vi "Autonomous Independent.vi"   [LabVIEW 2014]
doc: "This VI is called when autonomous begins, and will automatically be terminated when autonomous ends. You can carry out timed or sensor driven robot movement independently without needing to return to the caller."
uses:
  <vilib>/Rock Robotics/WPI/Joystick/WPI_JoystickGetSetRefNum.vi
  <vilib>/Rock Robotics/Network Tables/SD Write Numeric Array.vi
  Robot Global Data.vi
  <vilib>/addons/control/pid/pid.llb/PID (DBL).vi
  navX-MXP Library/navX-MXP IMU.lvlib
  <vilib>/addons/control/pid/NI_PID_pid.lvlib
panel:
  # "Be sure to right-click and choose Data Operations>>Make Current Value default if you want to save the array values with the VI"
types:
  T1 = cluster{"proportional gain (Kc)":dbl, "integral time (Ti, min)":dbl, "derivative time (Td, min)":dbl}
  T2 = typedef "WPI_JoystickDevRef.ctl" = cluster{"Device":T3}
  T3 = typedef "WPI_JoystickDeviceEnum.ctl" = enum16{"USB 0", "USB 1", "USB 2", "USB 3", "USB 4", "USB 5"}
  T4 = enum16{"centered", "deg0", "deg45", "deg90", "deg135", "deg180", "deg225", "deg270", "deg315"}
  T5 = typedef "WPI_MotorControlDeviceRef.ctl" = cluster{"DeviceStatus":errorcluster, "Type":T6, "PWM":cluster{"Controller":T7, "PWM Channel":T8, "DeadBand":T9}, "CAN":cluster{"Device Number":u8, "Control Mode":T10, "Semaphore":T11, "Max Vout":dbl, "TalonSRX Control Mode":T12}, "Invert":bool, "TransformRef":T13, "InvTransformRef":T13}
  T6 = typedef "WPI_MotorControlType.ctl" = enum16{"PWM", "CAN", "CANTalonSRX"}
  T7 = typedef "FPGA_TypedefDigitalModule.ctl" = enum16{"Controller 1"}
  T8 = typedef "FPGA_DIOPWMChannel.ctl" = enum8{"PWM 0", "PWM 1", "PWM 2", "PWM 3", "PWM 4", "PWM 5", "PWM 6", "PWM 7", "PWM 8", "PWM 9", "PWM MXP 0", "PWM MXP 1", "PWM MXP 2", "PWM MXP 3", "PWM MXP 4", "PWM MXP 5", "PWM MXP 6", "PWM MXP 7", "PWM MXP 8", "PWM MXP 9", "Invalid"}
  T9 = typedef "WPI_PWMDeadband.ctl" = cluster{"Name":string, "maxPositivePwm":i32, "minPositivePwm":i32, "centerPwm":i32, "maxNegativePwm":i32, "minNegativePwm":i32, "angularRange":u16}
  T10 = typedef "WPI_CANJaguar_ControlMode.ctl" = enum8{"Percent VBus", "Current", "Speed", "Position", "Voltage"}
  T11 = typedef "Semaphore RefNum" = refnum<k1>
  T12 = typedef "WPI_CANTalonSRX_APIControlMode.ctl" = enum8{"Percent VBus", "Speed", "Position", "Slave", "Unchanged / Invalid"}
  T13 = typedef "WPI_PWMTransform_ConPane.ctl" = refnum<vi>
  T14 = typedef "navX-MXP IMU.lvlib/navX Device TypeDef.ctl" = cluster{"navX Interface Protocol":T15, "navX Interface Protocol TypeDefs":cluster{"SPIDevRef":T16, "I2CDevRef":T18}, "navX System Information":cluster{"Board Information":T20, "Status":T21, "Offsets":T25}, "navX Common Information":cluster{"Update Rate (4Hz-60Hz)":T26, "refnum name":string, "error":errorcluster}}
  T15 = typedef "navX-MXP IMU.lvlib/navX Interface Protocol.ctl" = enum16{"SPI", "I2C"}
  T16 = typedef "WPI_SPIDevRef.ctl" = cluster{"DevStatus":errorcluster, "Handle":i32, "Controller":T7, "SPI Bus":T17}
  T17 = typedef "spi_bus.ctl" = enum16{"SPI On-Board, CS0", "SPI On-Board, CS1", "SPI On-Board, CS2", "SPI On-Board, CS3", "SPI MXP", "Invalid"}
  T18 = typedef "WPI_I2CDevRef.ctl" = cluster{"DevStatus":errorcluster, "Controller":T7, "Device Address":u8, "Handle":i32, "I2C Bus":T19}
  T19 = typedef "i2c_bus.ctl" = enum16{"I2C On-Board", "I2C MXP", "Invalid"}
  T20 = typedef "navX-MXP IMU.lvlib/navX Board Information.ctl" = cluster{"WhoAmI (50 | 0x32)":u8, "Board Revision":u8, "Firmware Major Version":u8, "Firmware Minor Version":u8}
  T21 = typedef "navX-MXP IMU.lvlib/navX Status Data.ctl" = cluster{"Update Rate Hz":u8, "Accelerometer Full-Scale Range":u8, "Gyro Full-Scale Range":u16, "NAVX_OP_STATUS":T22, "NAVX_CAL_STATUS":T23, "NAVX_SELFTEST_STATUS":u8, "NAVX_SENSOR_STATUS":T24}
  T22 = typedef "navX-MXP IMU.lvlib/navX NAVX_OP_STATUS.ctl" = u8
  T23 = typedef "navX-MXP IMU.lvlib/navX NAVX_CAL_STATUS.ctl" = u8
  T24 = typedef "navX-MXP IMU.lvlib/navX NAVX_SENSOR_STATUS.ctl" = cluster{"MOVING":bool, "YAW_STABLE":bool, "MAG_DISTURBANCE":bool, "ALTITUDE_VALID":bool, "SEALEVEL_PRESS_SET":bool, "FUSED_HEADING_VALID":bool}
  T25 = typedef "navX-MXP IMU.lvlib/navX Offsets Data.ctl" = cluster{"Yaw":dbl, "Quat W":dbl, "Quat X":dbl, "Quat Y":dbl, "Quat Z":dbl}
  T26 = typedef "navX-MXP IMU.lvlib/navX Update Rate.ctl" = u8
  T27 = typedef "navX-MXP IMU.lvlib/navX YPRH Data.ctl" = cluster{"Yaw":dbl, "Pitch":dbl, "Roll":dbl, "Heading":dbl}
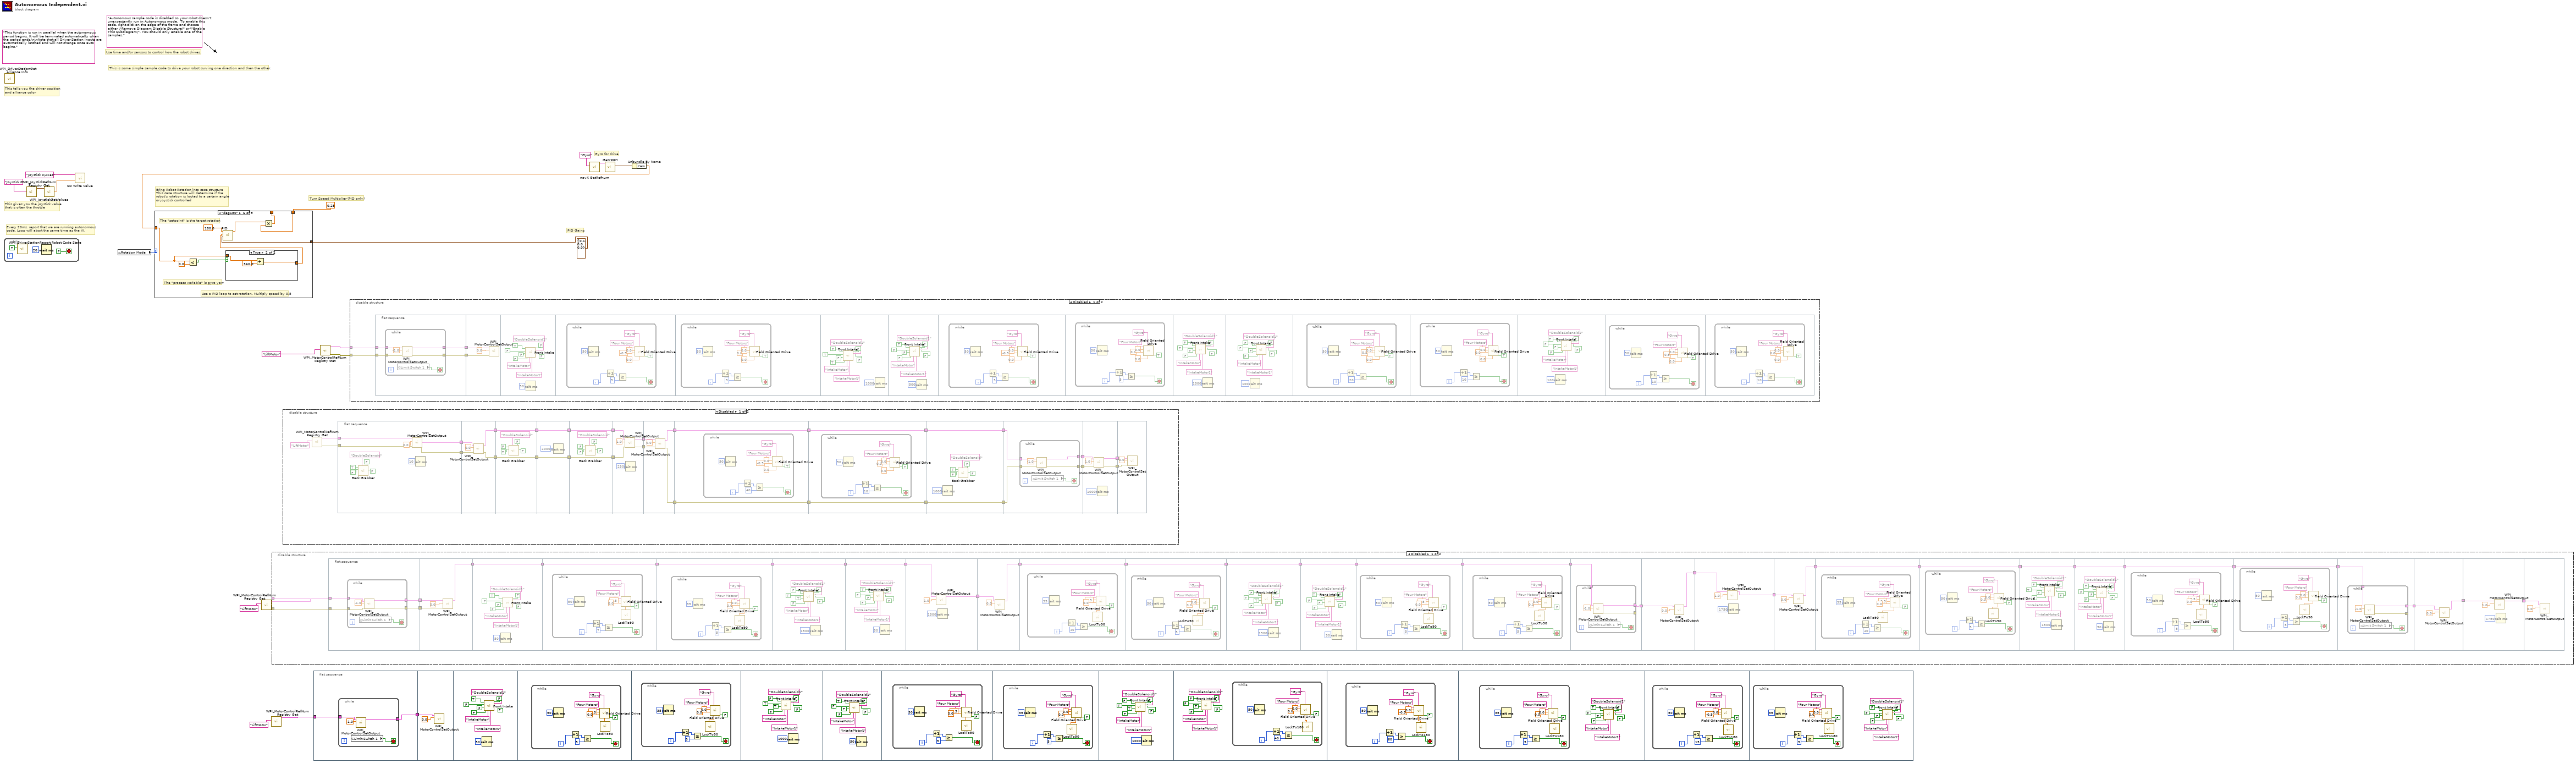
[diagram p0: block diagram]
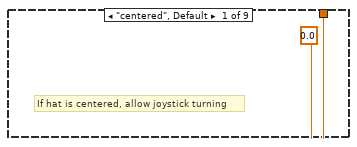
[diagram p5: hidden frame]
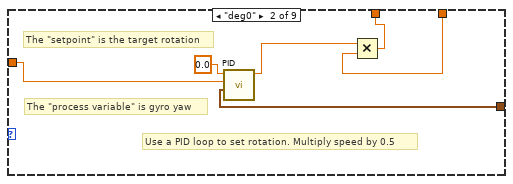
[diagram p6: hidden frame]
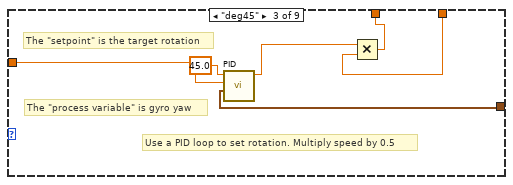
[diagram p7: hidden frame]
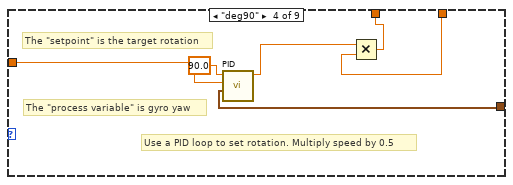
[diagram p8: hidden frame]
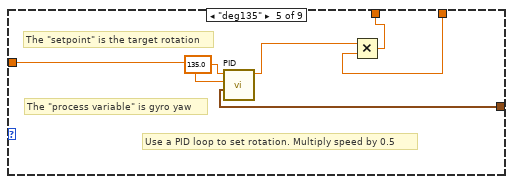
[diagram p9: hidden frame]
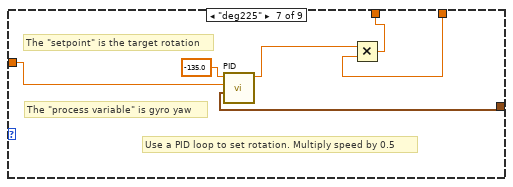
[diagram p11: hidden frame]
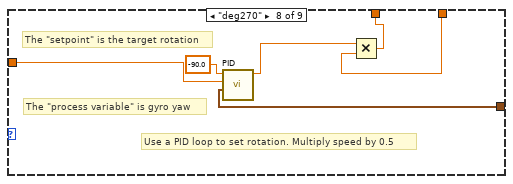
[diagram p12: hidden frame]
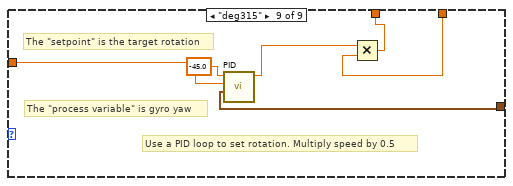
[diagram p13: hidden frame]
diagram:
  (unwired) "Autonomous sample code is disabled so your robot doesn't unexpectantly run in Autonomous mode.  To enable this code, right-click on the edge of the frame and choose either \"Remove Diagram Disable Structure\" or \"Enable This Subdiagram\". You should only enable one of the samples."
  (unwired) "This function is run in parallel when the autonomous period begins. It will be terminated automatically when the period ends.\n\nNote that all Driver Station inputs are automatically latched and will not change once auto begins."
  # "Turn Speed Multiplier (PID only)"
  # "PID Gains"
  # "Bring Robot Rotation into case structure\nThis case structure will determine if the \nrobot's rotation is locked to a certain angle\nor joystick controlled"
  # "Gyro for drive"
  # "This is some simple sample code to drive your robot curving one direction and then the other."
  # "Every 20ms, report that we are running autonomous\ncode. Loop will abort the same time as the VI."
  # "This gives you the joystick value\nthat is often the throttle"
  # "Use time and/or sensors to control how the robot drives."
  # "This tells you the driver position\nand alliance color"
  n1 = while {
    stop <- FALSE stop-if-true
    n2 = call <vilib>:"WPI_DriverStationReport Robot Code State.vi"("Autonomous"=TRUE) -> ()  [unwired: 10 in, 1 out]
    n3 = Wait (ms)(milliseconds to wait=u32 20) -> ()  [unwired: 1 out]
  }
  n4 = call <vilib>:"WPI_DriverStationGet Alliance Info.vi"() -> ()  [unwired: 12 out]
  n5 = call <vilib>:"WPI_JoystickRefNum Registry Get.vi"("refnum name"="Joystick 0") -> ("JoystickDevRef"=w19:T2)  [unwired: 1 in, 9 out]
  n6 = call <vilib>:"WPI_JoystickGetValues.vi"("JoystickDevRef"=w19) -> ("Axes"=w17:dbl[])  [unwired: 6 in, 4 out]
  n7 = call-poly <vilib>:"SD Write Value.vi"("Numeric Array"=w17, "Name"="Joystick 0/Axes") -> ()  [unwired: 8 in, 2 out]
  n8 = global read "Robot Global Data.vi" "Rotation Mode"() -> (w13:T4)
  n9 = call <vilib>:"WPI_MotorControlRefNum Registry Get.vi"("refnum name"="LiftMotor") -> ("error out"=w4:errorcluster, "MotorControlDevRef"=w5:T5)  [unwired: 9 in]
  n10 = call <vilib>:"WPI_MotorControlRefNum Registry Get.vi"("refnum name"="LiftMotor") -> ("MotorControlDevRef"=w2:T5)  [unwired: 9 in, 1 out]
  n11 = disable-structure shown="Disabled" {
    disable-tunnel: w5 -> [w25 _]
    disable-tunnel: w4 -> [w24 _]
    frame Disabled {
      n12 = flat-sequence {
        tunnel: w25 -> [w58]
        tunnel: w24 -> [w57]
        tunnel: [w56] -> w54
        tunnel: [w55] -> w53
        tunnel: w54 -> [w67]
        tunnel: w53 -> [w66]
        tunnel: [w65] -> w52
        tunnel: [w69] -> w51
        tunnel: w52 -> [w69]
        tunnel: [w79] -> w50
        tunnel: w51 -> [w79]
        tunnel: [w91] -> w49
        tunnel: w50 -> [w91]
        tunnel: [w103] -> w48
        tunnel: w49 -> [w103]
        tunnel: [w114] -> w47
        tunnel: w48 -> [w114]
        tunnel: w47 -> [w126]
        tunnel: [w125] -> w46
        tunnel: [w130] -> w45
        tunnel: w46 -> [w129]
        tunnel: [w132] -> w44
        tunnel: w45 -> [w132]
        tunnel: [w144] -> w43
        tunnel: w44 -> [w144]
        tunnel: [w156] -> w42
        tunnel: w43 -> [w156]
        tunnel: [w167] -> w41
        tunnel: w42 -> [w167]
        tunnel: [w178] -> w40
        tunnel: w41 -> [w178]
        tunnel: [w190] -> w39
        tunnel: w40 -> [w190]
        tunnel: w39 -> [w203]
        tunnel: [w202] -> w38
        tunnel: w38 -> [w210]
        tunnel: [w209] -> w37
        tunnel: w37 -> [w213]
        tunnel: [w212] -> w36
        tunnel: w36 -> [w217]
        tunnel: [w216] -> w35
        tunnel: [w219] -> w34
        tunnel: w35 -> [w219]
        tunnel: [w231] -> w33
        tunnel: w34 -> [w231]
        tunnel: [w243] -> w32
        tunnel: w33 -> [w243]
        tunnel: [w254] -> w31
        tunnel: w32 -> [w254]
        tunnel: [w265] -> w30
        tunnel: w31 -> [w265]
        tunnel: [w277] -> w29
        tunnel: w30 -> [w277]
        tunnel: w29 -> [w290]
        tunnel: [w289] -> w28
        tunnel: w28 -> [w297]
        tunnel: [w296] -> w27
        tunnel: w27 -> [w300]
        tunnel: [w299] -> w26
        tunnel: w26 -> [w303]
        frame #0 {
          n13 = while {
            tunnel: [w62] -> w56
            tunnel: [w61] -> w55
            tunnel: w58 -> [w60]
            tunnel: w57 -> [w59]
            stop <- w63 stop-if-true
            n14 = global read "Robot Global Data.vi" "Limit Switch 1"() -> (w63:bool)
            n15 = call <vilib>:"WPI_MotorControlSetOutput.vi"("error in (no error)"=w59, "Output"=-1.0, "MotorControlDevRef"=w60) -> ("error out"=w61:errorcluster, "MotorControlDevRef"=w62:T5)  [unwired: 6 in, 1 out]
          }
        }
        frame #1 {
          n16 = call <vilib>:"WPI_MotorControlSetOutput.vi"("error in (no error)"=w66, "Output"=0.0, "MotorControlDevRef"=w67) -> ("MotorControlDevRef"=w65:T5)  [unwired: 6 in, 2 out]
        }
        frame #2 {
          (unwired) FALSE ("Launchpad Button Backward")
          n17 = Wait (ms)(milliseconds to wait=u32 50) -> ()  [unwired: 1 out]
          n18 = call "Front Intake.vi"("Launchpad Button Backward"=FALSE, "Intake Motor 2 Refnum Name"="IntakeMotor1", "Intake Motor 1 Refnum Name"="IntakeMotor", "Solenoid Refnum Name"="DoubleSolenoid1", "Joystick Button Spin"=FALSE, "Joystick Button In"=FALSE, "Joystick Button Backward"=FALSE, "Joystick Button Forward"=TRUE) -> ()  [unwired: 4 in]
        }
        frame #3 {
          n19 = while {
            i -> [w90]
            stop <- w81 stop-if-true
            n20 = Wait (ms)(milliseconds to wait=u32 50) -> ()  [unwired: 1 out]
            n21 = Increment(x=w90) -> (x+1=w89:i32)
            n22 = Greater Or Equal?(x=w89, y=7) -> (x >= y?=w81:bool)
            n23 = call "LockTo90.vi"() -> ("rotation"=w80:dbl)  [unwired: 11 in]
            n24 = call "Field Oriented Drive.vi"("FIeld Oriented Drive Toggle Button"=FALSE, "Joystick Z Output"=w80, "Gyro Refnum Name"="Gyro", "Joystick Y Output"=0.0, "Joystick X Output"=-0.5, "Motor Refnum Name"="Four Motors") -> ()  [unwired: 6 in]
          }
        }
        frame #4 {
          n25 = while {
            i -> [w102]
            stop <- w93 stop-if-true
            n26 = Wait (ms)(milliseconds to wait=u32 35) -> ()  [unwired: 1 out]
            n27 = Increment(x=w102) -> (x+1=w101:i32)
            n28 = Greater Or Equal?(x=w101, y=5) -> (x >= y?=w93:bool)
            n29 = call "LockTo90.vi"() -> ("rotation"=w92:dbl)  [unwired: 11 in]
            n30 = call "Field Oriented Drive.vi"("FIeld Oriented Drive Toggle Button"=FALSE, "Joystick Z Output"=w92, "Gyro Refnum Name"="Gyro", "Joystick Y Output"=0.0, "Joystick X Output"=0.0, "Motor Refnum Name"="Four Motors") -> ()  [unwired: 6 in]
          }
        }
        frame #5 {
          n31 = call "Front Intake.vi"("Launchpad Button Backward"=FALSE, "Launchpad Button Forward"=FALSE ("Launchpad Button Backward"), "Intake Motor 2 Refnum Name"="IntakeMotor1", "Intake Motor 1 Refnum Name"="IntakeMotor", "Solenoid Refnum Name"="DoubleSolenoid1", "Joystick Button Spin"=FALSE, "Joystick Button In"=TRUE, "Joystick Button Backward"=TRUE, "Joystick Button Forward"=FALSE) -> ()  [unwired: 3 in]
          n32 = Wait (ms)(milliseconds to wait=u32 1500) -> ()  [unwired: 1 out]
        }
        frame #6 {
          n33 = call "Front Intake.vi"("Launchpad Button Backward"=FALSE, "Launchpad Button Forward"=FALSE ("Launchpad Button Backward"), "Intake Motor 2 Refnum Name"="IntakeMotor1", "Intake Motor 1 Refnum Name"="IntakeMotor", "Solenoid Refnum Name"="DoubleSolenoid1", "Joystick Button Spin"=FALSE, "Joystick Button In"=FALSE, "Joystick Button Backward"=FALSE, "Joystick Button Forward"=TRUE) -> ()  [unwired: 3 in]
          n34 = Wait (ms)(milliseconds to wait=u32 50) -> ()  [unwired: 1 out]
        }
        frame #7 {
          n35 = call <vilib>:"WPI_MotorControlSetOutput.vi"("Output"=1.0, "MotorControlDevRef"=w126) -> ("MotorControlDevRef"=w125:T5)  [unwired: 7 in, 2 out]
          n36 = Wait (ms)(milliseconds to wait=u32 1500) -> ()  [unwired: 1 out]
        }
        frame #8 {
          n37 = call <vilib>:"WPI_MotorControlSetOutput.vi"("Output"=0.0, "MotorControlDevRef"=w129) -> ("MotorControlDevRef"=w130:T5)  [unwired: 7 in, 2 out]
        }
        frame #9 {
          n38 = while {
            i -> [w143]
            stop <- w134 stop-if-true
            n39 = Wait (ms)(milliseconds to wait=u32 35) -> ()  [unwired: 1 out]
            n40 = Increment(x=w143) -> (x+1=w142:i32)
            n41 = Greater Or Equal?(x=w142, y=40) -> (x >= y?=w134:bool)
            n42 = call "LockTo90.vi"() -> ("rotation"=w133:dbl)  [unwired: 11 in]
            n43 = call "Field Oriented Drive.vi"("FIeld Oriented Drive Toggle Button"=FALSE, "Joystick Z Output"=w133, "Gyro Refnum Name"="Gyro", "Joystick Y Output"=0.0, "Joystick X Output"=-0.5, "Motor Refnum Name"="Four Motors") -> ()  [unwired: 6 in]
          }
        }
        frame #10 {
          n44 = while {
            i -> [w155]
            stop <- w146 stop-if-true
            n45 = Wait (ms)(milliseconds to wait=u32 50) -> ()  [unwired: 1 out]
            n46 = Increment(x=w155) -> (x+1=w154:i32)
            n47 = Greater Or Equal?(x=w154, y=5) -> (x >= y?=w146:bool)
            n48 = call "LockTo90.vi"() -> ("rotation"=w145:dbl)  [unwired: 11 in]
            n49 = call "Field Oriented Drive.vi"("FIeld Oriented Drive Toggle Button"=FALSE, "Joystick Z Output"=w145, "Gyro Refnum Name"="Gyro", "Joystick Y Output"=0.0, "Joystick X Output"=0.0, "Motor Refnum Name"="Four Motors") -> ()  [unwired: 6 in]
          }
        }
        frame #11 {
          n50 = call "Front Intake.vi"("Launchpad Button Backward"=FALSE, "Launchpad Button Forward"=FALSE ("Launchpad Button Backward"), "Intake Motor 2 Refnum Name"="IntakeMotor1", "Intake Motor 1 Refnum Name"="IntakeMotor", "Solenoid Refnum Name"="DoubleSolenoid1", "Joystick Button Spin"=FALSE, "Joystick Button In"=TRUE, "Joystick Button Backward"=TRUE, "Joystick Button Forward"=FALSE) -> ()  [unwired: 3 in]
          n51 = Wait (ms)(milliseconds to wait=u32 1500) -> ()  [unwired: 1 out]
        }
        frame #12 {
          n52 = call "Front Intake.vi"("Launchpad Button Backward"=FALSE, "Launchpad Button Forward"=FALSE ("Launchpad Button Backward"), "Intake Motor 2 Refnum Name"="IntakeMotor1", "Intake Motor 1 Refnum Name"="IntakeMotor", "Solenoid Refnum Name"="DoubleSolenoid1", "Joystick Button Spin"=FALSE, "Joystick Button In"=FALSE, "Joystick Button Backward"=FALSE, "Joystick Button Forward"=TRUE) -> ()  [unwired: 3 in]
          n53 = Wait (ms)(milliseconds to wait=u32 50) -> ()  [unwired: 1 out]
        }
        frame #13 {
          n54 = while {
            i -> [w189]
            stop <- w180 stop-if-true
            n55 = Wait (ms)(milliseconds to wait=u32 50) -> ()  [unwired: 1 out]
            n56 = Increment(x=w189) -> (x+1=w188:i32)
            n57 = Greater Or Equal?(x=w188, y=5) -> (x >= y?=w180:bool)
            n58 = call "LockTo90.vi"() -> ("rotation"=w179:dbl)  [unwired: 11 in]
            n59 = call "Field Oriented Drive.vi"("FIeld Oriented Drive Toggle Button"=FALSE, "Joystick Z Output"=w179, "Gyro Refnum Name"="Gyro", "Joystick Y Output"=0.0, "Joystick X Output"=-0.5, "Motor Refnum Name"="Four Motors") -> ()  [unwired: 6 in]
          }
        }
        frame #14 {
          n60 = while {
            i -> [w201]
            stop <- w192 stop-if-true
            n61 = Wait (ms)(milliseconds to wait=u32 50) -> ()  [unwired: 1 out]
            n62 = Increment(x=w201) -> (x+1=w200:i32)
            n63 = Greater Or Equal?(x=w200, y=5) -> (x >= y?=w192:bool)
            n64 = call "LockTo90.vi"() -> ("rotation"=w191:dbl)  [unwired: 11 in]
            n65 = call "Field Oriented Drive.vi"("FIeld Oriented Drive Toggle Button"=FALSE, "Joystick Z Output"=w191, "Gyro Refnum Name"="Gyro", "Joystick Y Output"=0.0, "Joystick X Output"=0.0, "Motor Refnum Name"="Four Motors") -> ()  [unwired: 6 in]
          }
        }
        frame #15 {
          n66 = while {
            tunnel: [w206] -> w202
            tunnel: [w205] -> _
            tunnel: w203 -> [w204]
            stop <- w207 stop-if-true
            n67 = global read "Robot Global Data.vi" "Limit Switch 1"() -> (w207:bool)
            n68 = call <vilib>:"WPI_MotorControlSetOutput.vi"("Output"=-1.0, "MotorControlDevRef"=w204) -> ("error out"=w205:errorcluster, "MotorControlDevRef"=w206:T5)  [unwired: 7 in, 1 out]
          }
        }
        frame #16 {
          n69 = call <vilib>:"WPI_MotorControlSetOutput.vi"("Output"=0.0, "MotorControlDevRef"=w210) -> ("MotorControlDevRef"=w209:T5)  [unwired: 7 in, 2 out]
        }
        frame #17 {
          n70 = call <vilib>:"WPI_MotorControlSetOutput.vi"("Output"=1.0, "MotorControlDevRef"=w213) -> ("MotorControlDevRef"=w212:T5)  [unwired: 7 in, 2 out]
          n71 = Wait (ms)(milliseconds to wait=u32 1750) -> ()  [unwired: 1 out]
        }
        frame #18 {
          n72 = call <vilib>:"WPI_MotorControlSetOutput.vi"("Output"=0.0, "MotorControlDevRef"=w217) -> ("MotorControlDevRef"=w216:T5)  [unwired: 7 in, 2 out]
        }
        frame #19 {
          n73 = while {
            i -> [w230]
            stop <- w221 stop-if-true
            n74 = Wait (ms)(milliseconds to wait=u32 35) -> ()  [unwired: 1 out]
            n75 = Increment(x=w230) -> (x+1=w229:i32)
            n76 = Greater Or Equal?(x=w229, y=40) -> (x >= y?=w221:bool)
            n77 = call "LockTo90.vi"() -> ("rotation"=w220:dbl)  [unwired: 11 in]
            n78 = call "Field Oriented Drive.vi"("FIeld Oriented Drive Toggle Button"=FALSE, "Joystick Z Output"=w220, "Gyro Refnum Name"="Gyro", "Joystick Y Output"=0.0, "Joystick X Output"=-0.5, "Motor Refnum Name"="Four Motors") -> ()  [unwired: 6 in]
          }
        }
        frame #20 {
          n79 = while {
            i -> [w242]
            stop <- w233 stop-if-true
            n80 = Wait (ms)(milliseconds to wait=u32 50) -> ()  [unwired: 1 out]
            n81 = Increment(x=w242) -> (x+1=w241:i32)
            n82 = Greater Or Equal?(x=w241, y=5) -> (x >= y?=w233:bool)
            n83 = call "LockTo90.vi"() -> ("rotation"=w232:dbl)  [unwired: 11 in]
            n84 = call "Field Oriented Drive.vi"("FIeld Oriented Drive Toggle Button"=FALSE, "Joystick Z Output"=w232, "Gyro Refnum Name"="Gyro", "Joystick Y Output"=0.0, "Joystick X Output"=0.0, "Motor Refnum Name"="Four Motors") -> ()  [unwired: 6 in]
          }
        }
        frame #21 {
          n85 = call "Front Intake.vi"("Launchpad Button Backward"=FALSE, "Launchpad Button Forward"=FALSE ("Launchpad Button Backward"), "Intake Motor 2 Refnum Name"="IntakeMotor1", "Intake Motor 1 Refnum Name"="IntakeMotor", "Solenoid Refnum Name"="DoubleSolenoid1", "Joystick Button Spin"=FALSE, "Joystick Button In"=TRUE, "Joystick Button Backward"=TRUE, "Joystick Button Forward"=FALSE) -> ()  [unwired: 3 in]
          n86 = Wait (ms)(milliseconds to wait=u32 1500) -> ()  [unwired: 1 out]
        }
        frame #22 {
          n87 = call "Front Intake.vi"("Launchpad Button Backward"=FALSE, "Launchpad Button Forward"=FALSE ("Launchpad Button Backward"), "Intake Motor 2 Refnum Name"="IntakeMotor1", "Intake Motor 1 Refnum Name"="IntakeMotor", "Solenoid Refnum Name"="DoubleSolenoid1", "Joystick Button Spin"=FALSE, "Joystick Button In"=FALSE, "Joystick Button Backward"=FALSE, "Joystick Button Forward"=TRUE) -> ()  [unwired: 3 in]
          n88 = Wait (ms)(milliseconds to wait=u32 50) -> ()  [unwired: 1 out]
        }
        frame #23 {
          n89 = while {
            i -> [w276]
            stop <- w267 stop-if-true
            n90 = Wait (ms)(milliseconds to wait=u32 50) -> ()  [unwired: 1 out]
            n91 = Increment(x=w276) -> (x+1=w275:i32)
            n92 = Greater Or Equal?(x=w275, y=5) -> (x >= y?=w267:bool)
            n93 = call "LockTo90.vi"() -> ("rotation"=w266:dbl)  [unwired: 11 in]
            n94 = call "Field Oriented Drive.vi"("FIeld Oriented Drive Toggle Button"=FALSE, "Joystick Z Output"=w266, "Gyro Refnum Name"="Gyro", "Joystick Y Output"=0.0, "Joystick X Output"=-0.5, "Motor Refnum Name"="Four Motors") -> ()  [unwired: 6 in]
          }
        }
        frame #24 {
          n95 = while {
            i -> [w288]
            stop <- w279 stop-if-true
            n96 = Wait (ms)(milliseconds to wait=u32 50) -> ()  [unwired: 1 out]
            n97 = Increment(x=w288) -> (x+1=w287:i32)
            n98 = Greater Or Equal?(x=w287, y=5) -> (x >= y?=w279:bool)
            n99 = call "LockTo90.vi"() -> ("rotation"=w278:dbl)  [unwired: 11 in]
            n100 = call "Field Oriented Drive.vi"("FIeld Oriented Drive Toggle Button"=FALSE, "Joystick Z Output"=w278, "Gyro Refnum Name"="Gyro", "Joystick Y Output"=0.0, "Joystick X Output"=0.0, "Motor Refnum Name"="Four Motors") -> ()  [unwired: 6 in]
          }
        }
        frame #25 {
          n101 = while {
            tunnel: [w293] -> w289
            tunnel: [w292] -> _
            tunnel: w290 -> [w291]
            stop <- w294 stop-if-true
            n102 = global read "Robot Global Data.vi" "Limit Switch 1"() -> (w294:bool)
            n103 = call <vilib>:"WPI_MotorControlSetOutput.vi"("Output"=-1.0, "MotorControlDevRef"=w291) -> ("error out"=w292:errorcluster, "MotorControlDevRef"=w293:T5)  [unwired: 7 in, 1 out]
          }
        }
        frame #26 {
          n104 = call <vilib>:"WPI_MotorControlSetOutput.vi"("Output"=0.0, "MotorControlDevRef"=w297) -> ("MotorControlDevRef"=w296:T5)  [unwired: 7 in, 2 out]
        }
        frame #27 {
          n105 = call <vilib>:"WPI_MotorControlSetOutput.vi"("Output"=1.0, "MotorControlDevRef"=w300) -> ("MotorControlDevRef"=w299:T5)  [unwired: 7 in, 2 out]
          n106 = Wait (ms)(milliseconds to wait=u32 1750) -> ()  [unwired: 1 out]
        }
        frame #28 {
          n107 = call <vilib>:"WPI_MotorControlSetOutput.vi"("Output"=0.0, "MotorControlDevRef"=w303) -> ()  [unwired: 7 in, 3 out]
        }
      }
    }
    frame Enabled {
    }
  }
  n108 = disable-structure shown="Disabled" {
    frame Disabled {
      n109 = call <vilib>:"WPI_MotorControlRefNum Registry Get.vi"("refnum name"="LiftMotor") -> ("error out"=w307:errorcluster, "MotorControlDevRef"=w305:T5)  [unwired: 9 in]
      n110 = flat-sequence {
        tunnel: [w335] -> w331
        tunnel: [w334] -> w330
        tunnel: w307 -> [w333]
        tunnel: w305 -> [w332]
        tunnel: [w346] -> w329
        tunnel: [w345] -> w328
        tunnel: w331 -> [w344]
        tunnel: w330 -> [w343]
        tunnel: [w349] -> w327
        tunnel: w329 -> [w349]
        tunnel: [w348] -> w326
        tunnel: w328 -> [w348]
        tunnel: [w356] -> w325
        tunnel: w327 -> [w356]
        tunnel: [w355] -> w324
        tunnel: w326 -> [w355]
        tunnel: [w359] -> w323
        tunnel: w325 -> [w359]
        tunnel: [w358] -> w322
        tunnel: w324 -> [w358]
        tunnel: w323 -> [w369]
        tunnel: w322 -> [w368]
        tunnel: [w366] -> w321
        tunnel: [w365] -> w320
        tunnel: w321 -> [w375]
        tunnel: w320 -> [w374]
        tunnel: [w372] -> w319
        tunnel: [w371] -> w318
        tunnel: [w377] -> w317
        tunnel: w319 -> [w377]
        tunnel: [w376] -> w316
        tunnel: w318 -> [w376]
        tunnel: w317 -> [w390]
        tunnel: [w390] -> w315
        tunnel: w316 -> [w389]
        tunnel: [w389] -> w314
        tunnel: [w403] -> w313
        tunnel: w315 -> [w403]
        tunnel: [w402] -> w312
        tunnel: w314 -> [w402]
        tunnel: w313 -> [w413]
        tunnel: w312 -> [w412]
        tunnel: [w411] -> w311
        tunnel: [w410] -> w310
        tunnel: w311 -> [w423]
        tunnel: w310 -> [w422]
        tunnel: [w421] -> w309
        tunnel: [w420] -> w308
        tunnel: w309 -> [w428]
        tunnel: w308 -> [w427]
        frame #0 {
          n111 = call "Back Grabber.vi"("Launchpad Button 2"=FALSE, "Launchpad Button 1"=FALSE, "Solenoid Refnum Name"="DoubleSolenoid", "Joystick Button 2"=FALSE, "Joystick Button 1"=TRUE) -> ()  [unwired: 7 in]
          n112 = call <vilib>:"WPI_MotorControlSetOutput.vi"("error in (no error)"=w333, "Output"=0.0, "MotorControlDevRef"=w332) -> ("error out"=w335:errorcluster, "MotorControlDevRef"=w334:T5)  [unwired: 6 in, 1 out]
          n113 = Wait (ms)(milliseconds to wait=u32 10) -> ()  [unwired: 1 out]
        }
        frame #1 {
          n114 = call <vilib>:"WPI_MotorControlSetOutput.vi"("error in (no error)"=w344, "Output"=0.0, "MotorControlDevRef"=w343) -> ("error out"=w345:errorcluster, "MotorControlDevRef"=w346:T5)  [unwired: 6 in, 1 out]
        }
        frame #2 {
          n115 = call "Back Grabber.vi"("Launchpad Button 2"=FALSE, "Launchpad Button 1"=FALSE, "Solenoid Refnum Name"="DoubleSolenoid", "Joystick Button 2"=TRUE, "Joystick Button 1"=FALSE) -> ()  [unwired: 7 in]
        }
        frame #3 {
          n116 = Wait (ms)(milliseconds to wait=u32 2000) -> ()  [unwired: 1 out]
        }
        frame #4 {
          n117 = call "Back Grabber.vi"("Launchpad Button 2"=FALSE, "Launchpad Button 1"=FALSE, "Solenoid Refnum Name"="DoubleSolenoid", "Joystick Button 2"=FALSE, "Joystick Button 1"=FALSE) -> ()  [unwired: 7 in]
        }
        frame #5 {
          n118 = call <vilib>:"WPI_MotorControlSetOutput.vi"("error in (no error)"=w368, "Output"=1.0, "MotorControlDevRef"=w369) -> ("error out"=w365:errorcluster, "MotorControlDevRef"=w366:T5)  [unwired: 6 in, 1 out]
          n119 = Wait (ms)(milliseconds to wait=u32 250) -> ()  [unwired: 1 out]
        }
        frame #6 {
          n120 = call <vilib>:"WPI_MotorControlSetOutput.vi"("error in (no error)"=w374, "Output"=0.0, "MotorControlDevRef"=w375) -> ("error out"=w371:errorcluster, "MotorControlDevRef"=w372:T5)  [unwired: 6 in, 1 out]
        }
        frame #7 {
          n121 = while {
            i -> [w388]
            stop <- w378 stop-if-true
            n122 = Wait (ms)(milliseconds to wait=u32 50) -> ()  [unwired: 1 out]
            n123 = Increment(x=w388) -> (x+1=w387:i32)
            n124 = Greater Or Equal?(x=w387, y=40) -> (x >= y?=w378:bool)
            n125 = call "Field Oriented Drive.vi"("FIeld Oriented Drive Toggle Button"=TRUE, "Joystick Z Output"=0.0, "Gyro Refnum Name"="Gyro", "Joystick Y Output"=-0.5, "Joystick X Output"=0.0, "Motor Refnum Name"="Four Motors") -> ()  [unwired: 6 in]
          }
        }
        frame #8 {
          n126 = while {
            i -> [w401]
            stop <- w391 stop-if-true
            n127 = Wait (ms)(milliseconds to wait=u32 50) -> ()  [unwired: 1 out]
            n128 = Increment(x=w401) -> (x+1=w400:i32)
            n129 = Greater Or Equal?(x=w400, y=10) -> (x >= y?=w391:bool)
            n130 = call "Field Oriented Drive.vi"("FIeld Oriented Drive Toggle Button"=TRUE, "Joystick Z Output"=0.0, "Gyro Refnum Name"="Gyro", "Joystick Y Output"=0.0, "Joystick X Output"=0.0, "Motor Refnum Name"="Four Motors") -> ()  [unwired: 6 in]
          }
        }
        frame #9 {
          n131 = Wait (ms)(milliseconds to wait=u32 1000) -> ()  [unwired: 1 out]
          n132 = call "Back Grabber.vi"("Launchpad Button 2"=FALSE, "Launchpad Button 1"=FALSE, "Solenoid Refnum Name"="DoubleSolenoid", "Joystick Button 2"=FALSE, "Joystick Button 1"=TRUE) -> ()  [unwired: 7 in]
        }
        frame #10 {
          n133 = while {
            tunnel: w413 -> [w419]
            tunnel: w412 -> [w418]
            tunnel: [w415] -> w411
            tunnel: [w414] -> w410
            stop <- w416 stop-if-true
            n134 = global read "Robot Global Data.vi" "Limit Switch 1"() -> (w416:bool)
            n135 = call <vilib>:"WPI_MotorControlSetOutput.vi"("error in (no error)"=w418, "Output"=-1.0, "MotorControlDevRef"=w419) -> ("error out"=w414:errorcluster, "MotorControlDevRef"=w415:T5)  [unwired: 6 in, 1 out]
          }
        }
        frame #11 {
          n136 = call <vilib>:"WPI_MotorControlSetOutput.vi"("error in (no error)"=w422, "Output"=1.0, "MotorControlDevRef"=w423) -> ("error out"=w420:errorcluster, "MotorControlDevRef"=w421:T5)  [unwired: 6 in, 1 out]
          n137 = Wait (ms)(milliseconds to wait=u32 1000) -> ()  [unwired: 1 out]
        }
        frame #12 {
          n138 = call <vilib>:"WPI_MotorControlSetOutput.vi"("error in (no error)"=w427, "Output"=0.0, "MotorControlDevRef"=w428) -> ()  [unwired: 6 in, 3 out]
        }
      }
    }
    frame Enabled {
    }
  }
  n139 = flat-sequence {
    tunnel: w2 -> [w430]
    tunnel: [w429] -> w1
    tunnel: w1 -> [w435]
    frame #0 {
      n140 = while {
        tunnel: [w432] -> w429
        tunnel: w430 -> [w431]
        stop <- w433 stop-if-true
        n141 = global read "Robot Global Data.vi" "Limit Switch 1"() -> (w433:bool)
        n142 = call <vilib>:"WPI_MotorControlSetOutput.vi"("Output"=-1.0, "MotorControlDevRef"=w431) -> ("MotorControlDevRef"=w432:T5)  [unwired: 7 in, 2 out]
      }
    }
    frame #1 {
      n143 = call <vilib>:"WPI_MotorControlSetOutput.vi"("Output"=0.0, "MotorControlDevRef"=w435) -> ()  [unwired: 7 in, 3 out]
    }
    frame #2 {
      (unwired) FALSE ("Launchpad Button Backward")
      n144 = Wait (ms)(milliseconds to wait=u32 50) -> ()  [unwired: 1 out]
      n145 = call "Front Intake.vi"("Launchpad Button Backward"=FALSE, "Intake Motor 2 Refnum Name"="IntakeMotor1", "Intake Motor 1 Refnum Name"="IntakeMotor", "Solenoid Refnum Name"="DoubleSolenoid1", "Joystick Button Spin"=FALSE, "Joystick Button In"=FALSE, "Joystick Button Backward"=FALSE, "Joystick Button Forward"=TRUE) -> ()  [unwired: 4 in]
    }
    frame #3 {
      n146 = while {
        i -> [w456]
        stop <- w447 stop-if-true
        n147 = Wait (ms)(milliseconds to wait=u32 50) -> ()  [unwired: 1 out]
        n148 = Increment(x=w456) -> (x+1=w455:i32)
        n149 = Greater Or Equal?(x=w455, y=5) -> (x >= y?=w447:bool)
        n150 = call "LockTo90.vi"() -> ("rotation"=w446:dbl)  [unwired: 11 in]
        n151 = call "Field Oriented Drive.vi"("FIeld Oriented Drive Toggle Button"=FALSE, "Joystick Z Output"=w446, "Gyro Refnum Name"="Gyro", "Joystick Y Output"=0.0, "Joystick X Output"=-0.5, "Motor Refnum Name"="Four Motors") -> ()  [unwired: 6 in]
      }
    }
    frame #4 {
      n152 = while {
        i -> [w467]
        stop <- w458 stop-if-true
        n153 = Wait (ms)(milliseconds to wait=u32 35) -> ()  [unwired: 1 out]
        n154 = Increment(x=w467) -> (x+1=w466:i32)
        n155 = Greater Or Equal?(x=w466, y=5) -> (x >= y?=w458:bool)
        n156 = call "LockTo90.vi"() -> ("rotation"=w457:dbl)  [unwired: 11 in]
        n157 = call "Field Oriented Drive.vi"("FIeld Oriented Drive Toggle Button"=FALSE, "Joystick Z Output"=w457, "Gyro Refnum Name"="Gyro", "Joystick Y Output"=0.0, "Joystick X Output"=0.0, "Motor Refnum Name"="Four Motors") -> ()  [unwired: 6 in]
      }
    }
    frame #5 {
      n158 = call "Front Intake.vi"("Launchpad Button Backward"=FALSE, "Launchpad Button Forward"=FALSE ("Launchpad Button Backward"), "Intake Motor 2 Refnum Name"="IntakeMotor1", "Intake Motor 1 Refnum Name"="IntakeMotor", "Solenoid Refnum Name"="DoubleSolenoid1", "Joystick Button Spin"=FALSE, "Joystick Button In"=TRUE, "Joystick Button Backward"=TRUE, "Joystick Button Forward"=FALSE) -> ()  [unwired: 3 in]
      n159 = Wait (ms)(milliseconds to wait=u32 1000) -> ()  [unwired: 1 out]
    }
    frame #6 {
      n160 = call "Front Intake.vi"("Launchpad Button Backward"=FALSE, "Launchpad Button Forward"=FALSE ("Launchpad Button Backward"), "Intake Motor 2 Refnum Name"="IntakeMotor1", "Intake Motor 1 Refnum Name"="IntakeMotor", "Solenoid Refnum Name"="DoubleSolenoid1", "Joystick Button Spin"=FALSE, "Joystick Button In"=FALSE, "Joystick Button Backward"=FALSE, "Joystick Button Forward"=TRUE) -> ()  [unwired: 3 in]
      n161 = Wait (ms)(milliseconds to wait=u32 50) -> ()  [unwired: 1 out]
    }
    frame #7 {
      n162 = while {
        i -> [w498]
        stop <- w489 stop-if-true
        n163 = Wait (ms)(milliseconds to wait=u32 50) -> ()  [unwired: 1 out]
        n164 = Increment(x=w498) -> (x+1=w497:i32)
        n165 = Greater Or Equal?(x=w497, y=5) -> (x >= y?=w489:bool)
        n166 = call "LockTo90.vi"() -> ("rotation"=w488:dbl)  [unwired: 11 in]
        n167 = call "Field Oriented Drive.vi"("FIeld Oriented Drive Toggle Button"=FALSE, "Joystick Z Output"=w488, "Gyro Refnum Name"="Gyro", "Joystick Y Output"=0.0, "Joystick X Output"=-0.5, "Motor Refnum Name"="Four Motors") -> ()  [unwired: 6 in]
      }
    }
    frame #8 {
      n168 = while {
        i -> [w509]
        stop <- w500 stop-if-true
        n169 = Wait (ms)(milliseconds to wait=u32 35) -> ()  [unwired: 1 out]
        n170 = Increment(x=w509) -> (x+1=w508:i32)
        n171 = Greater Or Equal?(x=w508, y=5) -> (x >= y?=w500:bool)
        n172 = call "LockTo90.vi"() -> ("rotation"=w499:dbl)  [unwired: 11 in]
        n173 = call "Field Oriented Drive.vi"("FIeld Oriented Drive Toggle Button"=FALSE, "Joystick Z Output"=w499, "Gyro Refnum Name"="Gyro", "Joystick Y Output"=0.0, "Joystick X Output"=0.0, "Motor Refnum Name"="Four Motors") -> ()  [unwired: 6 in]
      }
    }
    frame #9 {
      n174 = call "Front Intake.vi"("Launchpad Button Backward"=FALSE, "Launchpad Button Forward"=FALSE ("Launchpad Button Backward"), "Intake Motor 2 Refnum Name"="IntakeMotor1", "Intake Motor 1 Refnum Name"="IntakeMotor", "Solenoid Refnum Name"="DoubleSolenoid1", "Joystick Button Spin"=FALSE, "Joystick Button In"=TRUE, "Joystick Button Backward"=TRUE, "Joystick Button Forward"=FALSE) -> ()  [unwired: 3 in]
      n175 = Wait (ms)(milliseconds to wait=u32 1000) -> ()  [unwired: 1 out]
    }
    frame #10 {
      n176 = call "Front Intake.vi"("Launchpad Button Backward"=FALSE, "Launchpad Button Forward"=FALSE ("Launchpad Button Backward"), "Intake Motor 2 Refnum Name"="IntakeMotor1", "Intake Motor 1 Refnum Name"="IntakeMotor", "Solenoid Refnum Name"="DoubleSolenoid1", "Joystick Button Spin"=FALSE, "Joystick Button In"=TRUE, "Joystick Button Backward"=FALSE, "Joystick Button Forward"=FALSE) -> ()  [unwired: 3 in]
      n177 = while {
        i -> [w539]
        stop <- w530 stop-if-true
        n178 = Wait (ms)(milliseconds to wait=u32 50) -> ()  [unwired: 1 out]
        n179 = Increment(x=w539) -> (x+1=w538:i32)
        n180 = Greater Or Equal?(x=w538, y=40) -> (x >= y?=w530:bool)
        n181 = call "LockTo180.vi"() -> ("rotation"=w529:dbl)  [unwired: 11 in]
        n182 = call "Field Oriented Drive.vi"("FIeld Oriented Drive Toggle Button"=FALSE, "Joystick Z Output"=w529, "Gyro Refnum Name"="Gyro", "Joystick Y Output"=0.0, "Joystick X Output"=0.0, "Motor Refnum Name"="Four Motors") -> ()  [unwired: 6 in]
      }
    }
    frame #11 {
      n183 = while {
        i -> [w550]
        stop <- w541 stop-if-true
        n184 = Wait (ms)(milliseconds to wait=u32 50) -> ()  [unwired: 1 out]
        n185 = Increment(x=w550) -> (x+1=w549:i32)
        n186 = Greater Or Equal?(x=w549, y=60) -> (x >= y?=w541:bool)
        n187 = call "LockTo180.vi"() -> ("rotation"=w540:dbl)  [unwired: 11 in]
        n188 = call "Field Oriented Drive.vi"("FIeld Oriented Drive Toggle Button"=FALSE, "Joystick Z Output"=w540, "Gyro Refnum Name"="Gyro", "Joystick Y Output"=-0.5, "Joystick X Output"=0.0, "Motor Refnum Name"="Four Motors") -> ()  [unwired: 6 in]
      }
    }
    frame #12 {
      n189 = while {
        i -> [w570]
        stop <- w561 stop-if-true
        n190 = Wait (ms)(milliseconds to wait=u32 35) -> ()  [unwired: 1 out]
        n191 = Increment(x=w570) -> (x+1=w569:i32)
        n192 = Greater Or Equal?(x=w569, y=5) -> (x >= y?=w561:bool)
        n193 = call "LockTo180.vi"() -> ("rotation"=w560:dbl)  [unwired: 11 in]
        n194 = call "Field Oriented Drive.vi"("FIeld Oriented Drive Toggle Button"=FALSE, "Joystick Z Output"=w560, "Gyro Refnum Name"="Gyro", "Joystick Y Output"=0.0, "Joystick X Output"=0.0, "Motor Refnum Name"="Four Motors") -> ()  [unwired: 6 in]
      }
      n195 = call "Front Intake.vi"("Launchpad Button Backward"=FALSE, "Launchpad Button Forward"=FALSE ("Launchpad Button Backward"), "Intake Motor 2 Refnum Name"="IntakeMotor1", "Intake Motor 1 Refnum Name"="IntakeMotor", "Solenoid Refnum Name"="DoubleSolenoid1", "Joystick Button Spin"=FALSE, "Joystick Button In"=TRUE, "Joystick Button Backward"=FALSE, "Joystick Button Forward"=TRUE) -> ()  [unwired: 3 in]
    }
    frame #13 {
      n196 = while {
        i -> [w581]
        stop <- w572 stop-if-true
        n197 = Wait (ms)(milliseconds to wait=u32 50) -> ()  [unwired: 1 out]
        n198 = Increment(x=w581) -> (x+1=w580:i32)
        n199 = Greater Or Equal?(x=w580, y=15) -> (x >= y?=w572:bool)
        n200 = call "LockTo180.vi"() -> ("rotation"=w571:dbl)  [unwired: 11 in]
        n201 = call "Field Oriented Drive.vi"("FIeld Oriented Drive Toggle Button"=FALSE, "Joystick Z Output"=w571, "Gyro Refnum Name"="Gyro", "Joystick Y Output"=-0.5, "Joystick X Output"=0.0, "Motor Refnum Name"="Four Motors") -> ()  [unwired: 6 in]
      }
    }
    frame #14 {
      n202 = while {
        i -> [w601]
        stop <- w592 stop-if-true
        n203 = Wait (ms)(milliseconds to wait=u32 35) -> ()  [unwired: 1 out]
        n204 = Increment(x=w601) -> (x+1=w600:i32)
        n205 = Greater Or Equal?(x=w600, y=5) -> (x >= y?=w592:bool)
        n206 = call "LockTo180.vi"() -> ("rotation"=w591:dbl)  [unwired: 11 in]
        n207 = call "Field Oriented Drive.vi"("FIeld Oriented Drive Toggle Button"=FALSE, "Joystick Z Output"=w591, "Gyro Refnum Name"="Gyro", "Joystick Y Output"=0.0, "Joystick X Output"=0.0, "Motor Refnum Name"="Four Motors") -> ()  [unwired: 6 in]
      }
      n208 = call "Front Intake.vi"("Launchpad Button Backward"=FALSE, "Launchpad Button Forward"=FALSE ("Launchpad Button Backward"), "Intake Motor 2 Refnum Name"="IntakeMotor1", "Intake Motor 1 Refnum Name"="IntakeMotor", "Solenoid Refnum Name"="DoubleSolenoid1", "Joystick Button Spin"=FALSE, "Joystick Button In"=FALSE, "Joystick Button Backward"=FALSE, "Joystick Button Forward"=FALSE) -> ()  [unwired: 3 in]
    }
  }
  n209 = call <vilib>:"WPI_MotorControlRefNum Registry Get.vi"("refnum name"="LiftMotor") -> ("error out"=w7:errorcluster, "MotorControlDevRef"=w8:T5)  [unwired: 9 in]
  n210 = disable-structure shown="Disabled" {
    disable-tunnel: w8 -> [w603 _]
    disable-tunnel: w7 -> [w602 _]
    frame Disabled {
      n211 = flat-sequence {
        tunnel: w603 -> [w609]
        tunnel: w602 -> [w608]
        tunnel: [w607] -> w605
        tunnel: [w606] -> w604
        tunnel: w605 -> [w617]
        tunnel: w604 -> [w616]
        frame #0 {
          n212 = while {
            tunnel: w609 -> [w615]
            tunnel: w608 -> [w614]
            tunnel: [w611] -> w607
            tunnel: [w610] -> w606
            stop <- w612 stop-if-true
            n213 = global read "Robot Global Data.vi" "Limit Switch 1"() -> (w612:bool)
            n214 = call <vilib>:"WPI_MotorControlSetOutput.vi"("error in (no error)"=w614, "Output"=-1.0, "MotorControlDevRef"=w615) -> ("error out"=w610:errorcluster, "MotorControlDevRef"=w611:T5)  [unwired: 6 in, 1 out]
          }
        }
        frame #1 {
          n215 = call <vilib>:"WPI_MotorControlSetOutput.vi"("error in (no error)"=w616, "Output"=0.0, "MotorControlDevRef"=w617) -> ()  [unwired: 6 in, 3 out]
        }
        frame #2 {
          (unwired) FALSE ("Launchpad Button Backward")
          n216 = call "Front Intake.vi"("Launchpad Button Backward"=FALSE, "Intake Motor 2 Refnum Name"="IntakeMotor1", "Intake Motor 1 Refnum Name"="IntakeMotor", "Solenoid Refnum Name"="DoubleSolenoid1", "Joystick Button Spin"=FALSE, "Joystick Button In"=FALSE, "Joystick Button Backward"=FALSE, "Joystick Button Forward"=TRUE) -> ()  [unwired: 4 in]
          n217 = Wait (ms)(milliseconds to wait=u32 50) -> ()  [unwired: 1 out]
        }
        frame #3 {
          n218 = while {
            i -> [w638]
            stop <- w628 stop-if-true
            n219 = Wait (ms)(milliseconds to wait=u32 50) -> ()  [unwired: 1 out]
            n220 = Increment(x=w638) -> (x+1=w637:i32)
            n221 = Greater Or Equal?(x=w637, y=5) -> (x >= y?=w628:bool)
            n222 = call "Field Oriented Drive.vi"("FIeld Oriented Drive Toggle Button"=TRUE, "Joystick Z Output"=0.0, "Gyro Refnum Name"="Gyro", "Joystick Y Output"=-0.5, "Joystick X Output"=0.0, "Motor Refnum Name"="Four Motors") -> ()  [unwired: 6 in]
          }
        }
        frame #4 {
          n223 = while {
            i -> [w649]
            stop <- w639 stop-if-true
            n224 = Wait (ms)(milliseconds to wait=u32 50) -> ()  [unwired: 1 out]
            n225 = Increment(x=w649) -> (x+1=w648:i32)
            n226 = Greater Or Equal?(x=w648, y=5) -> (x >= y?=w639:bool)
            n227 = call "Field Oriented Drive.vi"("FIeld Oriented Drive Toggle Button"=TRUE, "Joystick Z Output"=0.0, "Gyro Refnum Name"="Gyro", "Joystick Y Output"=0.0, "Joystick X Output"=0.0, "Motor Refnum Name"="Four Motors") -> ()  [unwired: 6 in]
          }
        }
        frame #5 {
          n228 = call "Front Intake.vi"("Launchpad Button Backward"=FALSE, "Launchpad Button Forward"=FALSE ("Launchpad Button Backward"), "Intake Motor 2 Refnum Name"="IntakeMotor1", "Intake Motor 1 Refnum Name"="IntakeMotor", "Solenoid Refnum Name"="DoubleSolenoid1", "Joystick Button Spin"=TRUE, "Joystick Button In"=FALSE, "Joystick Button Backward"=TRUE, "Joystick Button Forward"=FALSE) -> ()  [unwired: 3 in]
          n229 = Wait (ms)(milliseconds to wait=u32 1000) -> ()  [unwired: 1 out]
        }
        frame #6 {
          n230 = call "Front Intake.vi"("Launchpad Button Backward"=FALSE, "Launchpad Button Forward"=FALSE ("Launchpad Button Backward"), "Intake Motor 2 Refnum Name"="IntakeMotor1", "Intake Motor 1 Refnum Name"="IntakeMotor", "Solenoid Refnum Name"="DoubleSolenoid1", "Joystick Button Spin"=FALSE, "Joystick Button In"=FALSE, "Joystick Button Backward"=FALSE, "Joystick Button Forward"=TRUE) -> ()  [unwired: 3 in]
          n231 = Wait (ms)(milliseconds to wait=u32 500) -> ()  [unwired: 1 out]
        }
        frame #7 {
          n232 = while {
            i -> [w680]
            stop <- w670 stop-if-true
            n233 = Wait (ms)(milliseconds to wait=u32 50) -> ()  [unwired: 1 out]
            n234 = Increment(x=w680) -> (x+1=w679:i32)
            n235 = Greater Or Equal?(x=w679, y=5) -> (x >= y?=w670:bool)
            n236 = call "Field Oriented Drive.vi"("FIeld Oriented Drive Toggle Button"=TRUE, "Joystick Z Output"=0.0, "Gyro Refnum Name"="Gyro", "Joystick Y Output"=-0.5, "Joystick X Output"=0.0, "Motor Refnum Name"="Four Motors") -> ()  [unwired: 6 in]
          }
        }
        frame #8 {
          n237 = while {
            i -> [w691]
            stop <- w681 stop-if-true
            n238 = Wait (ms)(milliseconds to wait=u32 50) -> ()  [unwired: 1 out]
            n239 = Increment(x=w691) -> (x+1=w690:i32)
            n240 = Greater Or Equal?(x=w690, y=5) -> (x >= y?=w681:bool)
            n241 = call "Field Oriented Drive.vi"("FIeld Oriented Drive Toggle Button"=TRUE, "Joystick Z Output"=0.0, "Gyro Refnum Name"="Gyro", "Joystick Y Output"=0.0, "Joystick X Output"=0.0, "Motor Refnum Name"="Four Motors") -> ()  [unwired: 6 in]
          }
        }
        frame #9 {
          n242 = call "Front Intake.vi"("Launchpad Button Backward"=FALSE, "Launchpad Button Forward"=FALSE ("Launchpad Button Backward"), "Intake Motor 2 Refnum Name"="IntakeMotor1", "Intake Motor 1 Refnum Name"="IntakeMotor", "Solenoid Refnum Name"="DoubleSolenoid1", "Joystick Button Spin"=FALSE, "Joystick Button In"=TRUE, "Joystick Button Backward"=TRUE, "Joystick Button Forward"=FALSE) -> ()  [unwired: 3 in]
          n243 = Wait (ms)(milliseconds to wait=u32 1500) -> ()  [unwired: 1 out]
        }
        frame #10 {
          n244 = Wait (ms)(milliseconds to wait=u32 100) -> ()  [unwired: 1 out]
          n245 = call "Front Intake.vi"("Launchpad Button Backward"=FALSE, "Launchpad Button Forward"=FALSE ("Launchpad Button Backward"), "Intake Motor 2 Refnum Name"="IntakeMotor1", "Intake Motor 1 Refnum Name"="IntakeMotor", "Solenoid Refnum Name"="DoubleSolenoid1", "Joystick Button Spin"=FALSE, "Joystick Button In"=FALSE, "Joystick Button Backward"=FALSE, "Joystick Button Forward"=FALSE) -> ()  [unwired: 3 in]
        }
        frame #11 {
          n246 = while {
            i -> [w722]
            stop <- w712 stop-if-true
            n247 = Wait (ms)(milliseconds to wait=u32 50) -> ()  [unwired: 1 out]
            n248 = Increment(x=w722) -> (x+1=w721:i32)
            n249 = Greater Or Equal?(x=w721, y=20) -> (x >= y?=w712:bool)
            n250 = call "Field Oriented Drive.vi"("FIeld Oriented Drive Toggle Button"=TRUE, "Joystick Z Output"=0.0, "Gyro Refnum Name"="Gyro", "Joystick Y Output"=0.5, "Joystick X Output"=0.0, "Motor Refnum Name"="Four Motors") -> ()  [unwired: 6 in]
          }
        }
        frame #12 {
          n251 = while {
            i -> [w733]
            stop <- w723 stop-if-true
            n252 = Wait (ms)(milliseconds to wait=u32 50) -> ()  [unwired: 1 out]
            n253 = Increment(x=w733) -> (x+1=w732:i32)
            n254 = Greater Or Equal?(x=w732, y=10) -> (x >= y?=w723:bool)
            n255 = call "Field Oriented Drive.vi"("FIeld Oriented Drive Toggle Button"=TRUE, "Joystick Z Output"=0.0, "Gyro Refnum Name"="Gyro", "Joystick Y Output"=0.0, "Joystick X Output"=0.0, "Motor Refnum Name"="Four Motors") -> ()  [unwired: 6 in]
          }
        }
        frame #13 {
          n256 = Wait (ms)(milliseconds to wait=u32 100) -> ()  [unwired: 1 out]
          n257 = call "Front Intake.vi"("Launchpad Button Backward"=FALSE, "Launchpad Button Forward"=FALSE ("Launchpad Button Backward"), "Intake Motor 2 Refnum Name"="IntakeMotor1", "Intake Motor 1 Refnum Name"="IntakeMotor", "Solenoid Refnum Name"="DoubleSolenoid1", "Joystick Button Spin"=FALSE, "Joystick Button In"=FALSE, "Joystick Button Backward"=FALSE, "Joystick Button Forward"=TRUE) -> ()  [unwired: 3 in]
        }
        frame #14 {
          n258 = while {
            i -> [w754]
            stop <- w744 stop-if-true
            n259 = Wait (ms)(milliseconds to wait=u32 50) -> ()  [unwired: 1 out]
            n260 = Increment(x=w754) -> (x+1=w753:i32)
            n261 = Greater Or Equal?(x=w753, y=10) -> (x >= y?=w744:bool)
            n262 = call "Field Oriented Drive.vi"("FIeld Oriented Drive Toggle Button"=TRUE, "Joystick Z Output"=0.0, "Gyro Refnum Name"="Gyro", "Joystick Y Output"=0.5, "Joystick X Output"=0.0, "Motor Refnum Name"="Four Motors") -> ()  [unwired: 6 in]
          }
        }
        frame #15 {
          n263 = while {
            i -> [w765]
            stop <- w755 stop-if-true
            n264 = Wait (ms)(milliseconds to wait=u32 50) -> ()  [unwired: 1 out]
            n265 = Increment(x=w765) -> (x+1=w764:i32)
            n266 = Greater Or Equal?(x=w764, y=10) -> (x >= y?=w755:bool)
            n267 = call "Field Oriented Drive.vi"("FIeld Oriented Drive Toggle Button"=TRUE, "Joystick Z Output"=0.0, "Gyro Refnum Name"="Gyro", "Joystick Y Output"=0.0, "Joystick X Output"=0.0, "Motor Refnum Name"="Four Motors") -> ()  [unwired: 6 in]
          }
        }
      }
    }
    frame Enabled {
    }
  }
  n268 = call "navX GetRefnum.vi"("refnum name"="Gyro") -> ("navX Device TypeDef"=w16:T14)  [unwired: 9 in, 1 out]
  n269 = call "GetYPRH.vi"("navX Device TypeDef"=w16) -> ("YPRH"=w14:T27)  [unwired: 8 in, 2 out]
  n270 = Unbundle By Name(w14) -> ("Yaw"=w10:dbl)
  n271 = case shown="\"deg180\"" w13 {
    tunnel: [0.0 w768 w773 w779 w785 w791 w804 w810 w816] -> _
    tunnel: T1 {"proportional gain (Kc)"=0.1, "integral time (Ti, min)"=0.0, "derivative time (Td, min)"=0.0} ("PID gains") -> [_ w771 w776 w782 w788 w797 w807 w813 w818]
    tunnel: 0.25 -> [_ w769 w775 w781 w787 w796 w806 w812 w819]
    tunnel: w10 -> [_ w767 w774 w780 w786 w792 w805 w811 w817]
    frame "centered", Default {
      # "If hat is centered, allow joystick turning"
    }
    frame "deg0" {
      # "The \"setpoint\" is the target rotation"
      # "The \"process variable\" is gyro yaw"
      # "Use a PID loop to set rotation. Multiply speed by 0.5"
      n272 = call-poly <vilib>:"PID.vi"("PID gains"=w771, "process variable"=w767, "setpoint"=0.0) -> ("output"=w770:dbl)  [unwired: 7 in, 1 out]
      n273 = Multiply(x=w770, y=w769) -> (x*y=w768:dbl)
    }
    frame "deg45" {
      # "The \"setpoint\" is the target rotation"
      # "The \"process variable\" is gyro yaw"
      # "Use a PID loop to set rotation. Multiply speed by 0.5"
      n274 = call-poly <vilib>:"PID.vi"("PID gains"=w776, "process variable"=w774, "setpoint"=45.0) -> ("output"=w777:dbl)  [unwired: 7 in, 1 out]
      n275 = Multiply(x=w777, y=w775) -> (x*y=w773:dbl)
    }
    frame "deg90" {
      # "The \"setpoint\" is the target rotation"
      # "The \"process variable\" is gyro yaw"
      # "Use a PID loop to set rotation. Multiply speed by 0.5"
      n276 = call-poly <vilib>:"PID.vi"("PID gains"=w782, "process variable"=w780, "setpoint"=90.0) -> ("output"=w783:dbl)  [unwired: 7 in, 1 out]
      n277 = Multiply(x=w783, y=w781) -> (x*y=w779:dbl)
    }
    frame "deg135" {
      # "The \"setpoint\" is the target rotation"
      # "The \"process variable\" is gyro yaw"
      # "Use a PID loop to set rotation. Multiply speed by 0.5"
      n278 = call-poly <vilib>:"PID.vi"("PID gains"=w788, "process variable"=w786, "setpoint"=135.0) -> ("output"=w789:dbl)  [unwired: 7 in, 1 out]
      n279 = Multiply(x=w789, y=w787) -> (x*y=w785:dbl)
    }
    frame "deg180" {
      # "The \"setpoint\" is the target rotation"
      # "The \"process variable\" is gyro yaw"
      # "Use a PID loop to set rotation. Multiply speed by 0.5"
      n280 = Less?(x=w792, y=0.0) -> (x < y?=w793:bool)
      n281 = case shown="True" w793 {
        tunnel: w792 -> [w800 w803]
        tunnel: [w800 w801] -> w795
        frame False {
        }
        frame True {
          n282 = Add(x=w803, y=360.0) -> (x+y=w801:dbl)
        }
      }
      n283 = call-poly <vilib>:"PID.vi"("PID gains"=w797, "process variable"=w795, "setpoint"=180.0) -> ("output"=w798:dbl)  [unwired: 7 in, 1 out]
      n284 = Multiply(x=w798, y=w796) -> (x*y=w791:dbl)
    }
    frame "deg225" {
      # "The \"setpoint\" is the target rotation"
      # "The \"process variable\" is gyro yaw"
      # "Use a PID loop to set rotation. Multiply speed by 0.5"
      n285 = call-poly <vilib>:"PID.vi"("PID gains"=w807, "process variable"=w805, "setpoint"=-135.0) -> ("output"=w808:dbl)  [unwired: 7 in, 1 out]
      n286 = Multiply(x=w808, y=w806) -> (x*y=w804:dbl)
    }
    frame "deg270" {
      # "The \"setpoint\" is the target rotation"
      # "The \"process variable\" is gyro yaw"
      # "Use a PID loop to set rotation. Multiply speed by 0.5"
      n287 = call-poly <vilib>:"PID.vi"("PID gains"=w813, "process variable"=w811, "setpoint"=-90.0) -> ("output"=w814:dbl)  [unwired: 7 in, 1 out]
      n288 = Multiply(x=w814, y=w812) -> (x*y=w810:dbl)
    }
    frame "deg315" {
      # "The \"setpoint\" is the target rotation"
      # "The \"process variable\" is gyro yaw"
      # "Use a PID loop to set rotation. Multiply speed by 0.5"
      n289 = call-poly <vilib>:"PID.vi"("PID gains"=w818, "process variable"=w817, "setpoint"=-45.0) -> ("output"=w820:dbl)  [unwired: 7 in, 1 out]
      n290 = Multiply(x=w820, y=w819) -> (x*y=w816:dbl)
    }
  }
